vi "Read DI Faults.vi"() -> ()   [LabVIEW 2017]
panel:
  in  "stop":bool
  out "Faults":bool[](array[boolean])
  in  "Inputs":bool[](array[boolean])
  out "Live DI Data":u32[](array[numeric])
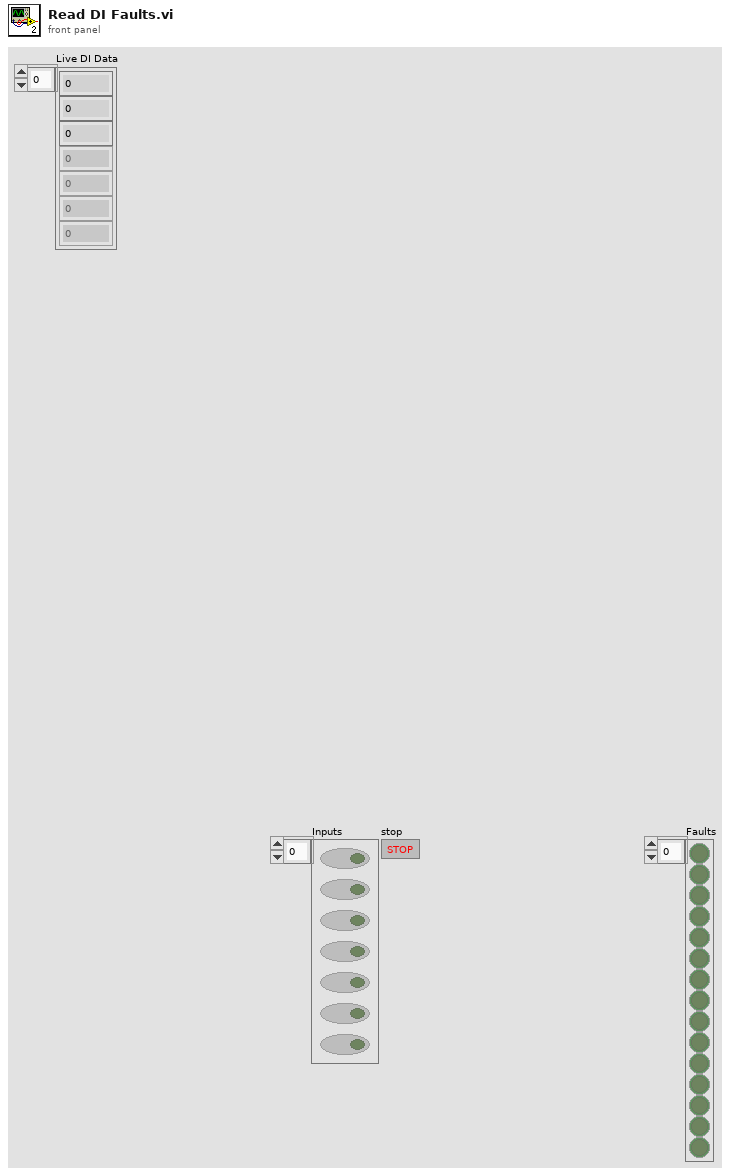
[diagram p1: front panel]
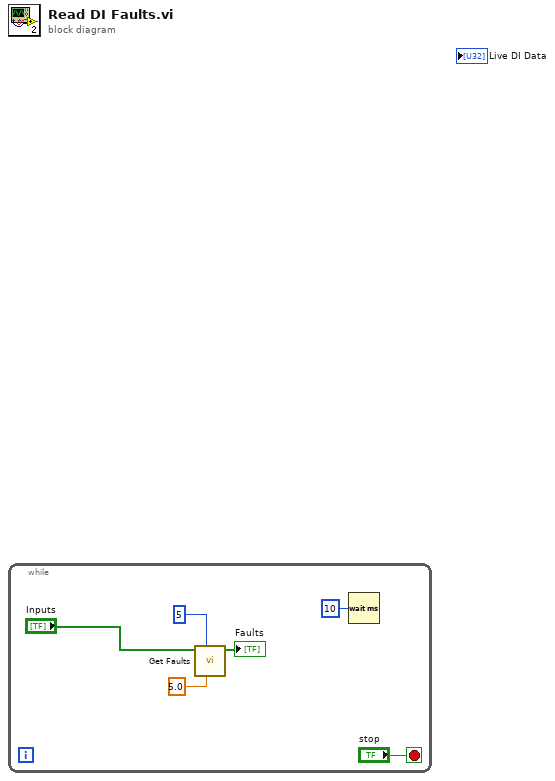
[diagram p0: block diagram]
diagram:
  n1 = while {
    stop <- "stop" stop-if-true
    n2 = call "Get Faults.vi"("Timer(Sec)"=5.0, "No of Inputs"=5, "Inputs"="Inputs") -> ("Faults"=→"Faults":bool[])  [unwired: 8 in]
    n3 = Wait (ms)(milliseconds to wait=u32 10) -> ()  [unwired: 1 out]
  }
